vi "Handle setAllData.vi"(8 "error in (no error)":errorcluster, 10 "AllData":variant, 11 "Inst.RP100 in":refnum<class "Inst.RP100.lvclass">) -> (0 "error out":errorcluster, 3 "Inst.RP100 out":refnum<class "Inst.RP100.lvclass">)   [LabVIEW 2019, in "Inst.RP100.lvlib" / "Inst.RP100.lvclass"]
doc: "Override to handle \"getAll\" or \"getAllData\" commands for <b>your</b> Instrument"
uses:
  Inst.RP100.lvclass
  Typedefs/Inst.RP100.getAll--Cluster.ctl
  Inst.RP100.lvclass/Inst.RP100.ctl
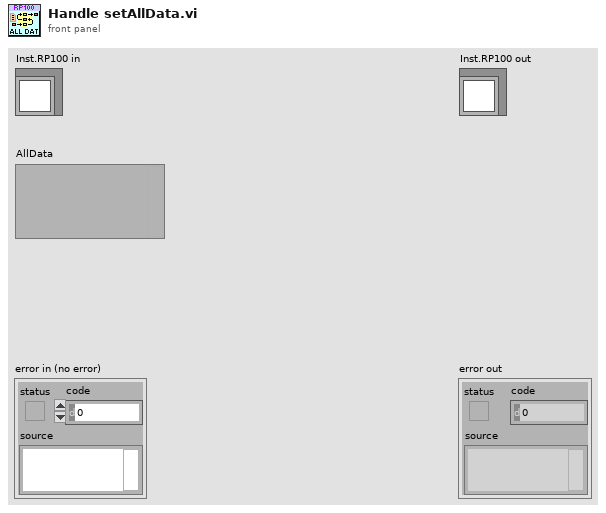
[diagram p1: front panel]
types:
  T1 = typedef "Inst.RP100.lvlib/Inst.RP100.lvclass/Inst.RP100.getAll--Cluster.ctl" = cluster{"OutputStateCh1":string, "OutputStateCh2":string, "LevelCh1":dbl, "LevelCh2":dbl, "SlewCh1":dbl, "SlewCh2":dbl, "MeasuredVCh1":dbl, "MeasuredVCh2":dbl, "MeasuredICh1":dbl, "MeasuredICh2":dbl}
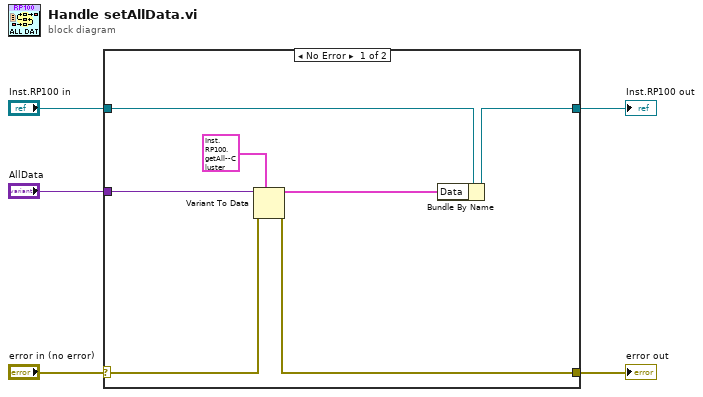
[diagram p0: block diagram]
diagram:
  n1 = case shown="No Error" "error in (no error)" {
    selector: "error in (no error)" -> [w7 w14]
    tunnel: [w6 w14] -> w5
    tunnel: [w9 w13] -> w4
    tunnel: "Inst.RP100 in" -> [w8 w13]
    tunnel: "AllData" -> [w10 _]
    frame No Error {
      n2 = Variant To Data(error in=w7, type=T1 {"OutputStateCh1"="", "OutputStateCh2"="", "LevelCh1"=0.0, "LevelCh2"=0.0, "SlewCh1"=0.0, "SlewCh2"=0.0, "MeasuredVCh1"=0.0, "MeasuredVCh2"=0.0, "MeasuredICh1"=0.0, "MeasuredICh2"=0.0} ("Data"), Variant=w10) -> (data=w12:T1, error out=w6:errorcluster)
      n3 = Bundle By Name(cluster=w8, "Data"=w12) -> (w9:refnum<class "Inst.RP100.lvclass">)
    }
    frame Error {
    }
  }
  "error out" <- w5
  "Inst.RP100 out" <- w4
